vi "LVIS_MsgPrompt.vi"(8 "Error In":errorcluster, 11 "Msg State":T1) -> (0 "Error Out":errorcluster)   [LabVIEW 2015]
doc: "User message prompt."
uses:
  Ctrls/LVIS_Msg State.ctl
  Globals/LVIS_DcGlobals.vi
panel:
  out "String":string
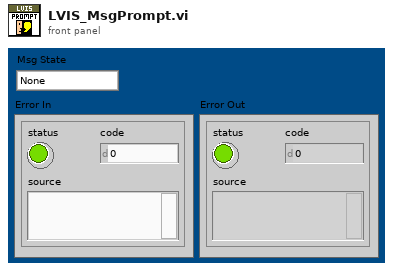
[diagram p1: front panel]
types:
  T1 = typedef "LVIS_Msg State.ctl" = enum16{"None", "Offline", "Online", "Backup Full"}
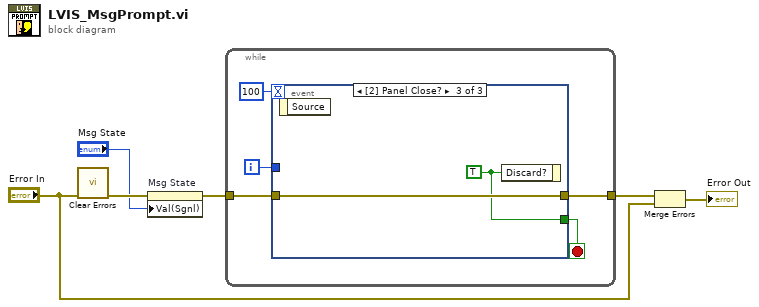
[diagram p0: block diagram]
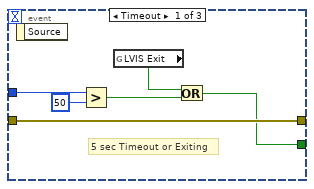
[diagram p2: hidden frame]
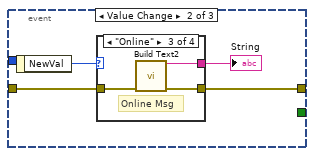
[diagram p3: hidden frame]
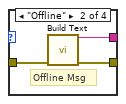
[diagram p5: hidden frame]
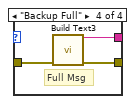
[diagram p6: hidden frame]
diagram:
  n1 = call <vilib>:"Clear Errors.vi"("error in (no error)"="Error In") -> ("error out"=w5:errorcluster)  [unwired: 5 in, 1 out]
  n2 = property on="Msg State" class="Enum (strict)"(error in=w5, "Val(Sgnl)"="Msg State") -> (error out=w6:errorcluster)  [unwired: 1 in, 1 out]
  n3 = while {
    tunnel: w6 -> [w11]
    tunnel: [w10] -> w4
    i -> [w8]
    stop <- w7 stop-if-true
    n4 = event shown="[2] Panel Close?" {
      selector: _ -> [_ _ _]
      dyn-events: _ -> [_ _ _]
      timeout: 100 -> [_ _ _]
      tunnel: w11 -> [w15 w21 w33]
      tunnel: [w15 w19 w33] -> w10
      tunnel: w8 -> [w17 _ _]
      tunnel: [w14 _ w32] -> w7
      event Timeout {
        # "5 sec Timeout or Exiting"
        n5 = event-data() -> ()  [unwired: 1 in, 1 out]
        n6 = Greater?(x=w17, y=50) -> (0:w12:bool)
        n7 = global read "LVIS_DcGlobals.vi" "LVIS Exit"() -> (w13:bool)
        n8 = Or(x=w13, y=w12) -> (x .or. y?=w14:bool)
      }
      event Value Change {
        n9 = event-data() -> ("NewVal"=w20:T1)  [unwired: 1 in]
        n10 = case shown="\"Online\"" w20 {
          tunnel: w21 -> [w22 w25 w28 w31]
          tunnel: [w22 w24 w27 w30] -> w19
          tunnel: [_ w23 w26 w29] -> w18
          frame "None", Default {
          }
          frame "Offline" {
            # "Offline Msg"
            n11 = call "Build Text"("error in (no error)"=w25) -> ("Result"=w23:string, "error out"=w24:errorcluster)  [unwired: 13 in]
          }
          frame "Online" {
            # "Online Msg"
            n12 = call "Build Text2"("error in (no error)"=w28) -> ("Result"=w26:string, "error out"=w27:errorcluster)  [unwired: 13 in]
          }
          frame "Backup Full" {
            # "Full Msg"
            n13 = call "Build Text3"("error in (no error)"=w31) -> ("Result"=w29:string, "error out"=w30:errorcluster)  [unwired: 13 in]
          }
        }
        "String" <- w18
      }
      event Panel Close? {
        w32 = TRUE ("Discard?")
        n14 = event-data() -> ()  [unwired: 1 in, 1 out]
        n15 = event-data("Discard?"=w32) -> ()  [unwired: 1 in, 1 out]
      }
    }
  }
  n16 = Merge Errors(w4, "Error In") -> (→"Error Out":errorcluster)
